vi "Update Actuator Setpoint.vi"(8 "error in (no error)":errorcluster, 11 "Model in":refnum<class "Model.lvclass">) -> (0 "error out":errorcluster, 3 "Model out":refnum<class "Model.lvclass">)   [LabVIEW 2015, in "Model.lvclass"]
uses:
  Model.lvclass
  Common_RT_FAILC/FAILC/FAILC.lvclass
  Modbus/DesktopModbus/DesktopModbus.lvclass
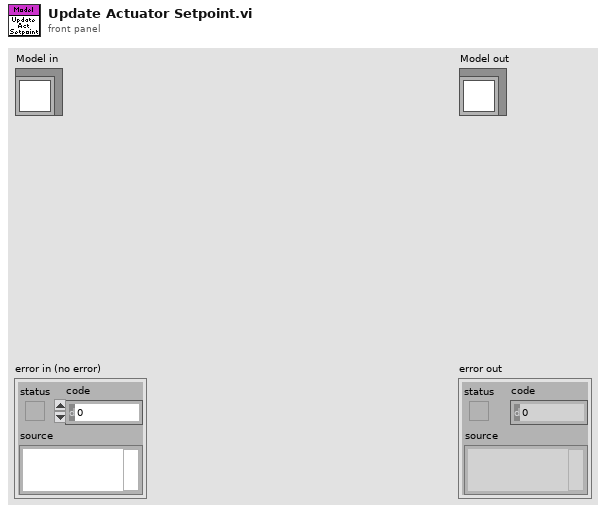
[diagram p1: front panel]
types:
  T1 = typedef "RTFAILC.lvlib/FAData.ctl" = cluster{"FAConstants":T2, "FACommand":T3, "FATelemetry":T5, "FAResponses":T6}
  T2 = typedef "RTFAILC.lvlib/FAConstants.ctl" = cluster{"ID":i16}
  T3 = typedef "RTFAILC.lvlib/FACommand.ctl" = cluster{"AxialSetPoint":i32, "LateralSetPoint":i32, "PressureServoValveSettings":T4, "BoosterValveSettings":T4}
  T4 = typedef "RTFAILC.lvlib/FAPID.ctl" = cluster{"Kp":sgl, "Ki":sgl, "Kd":sgl, "Kf":sgl}
  T5 = typedef "RTFAILC.lvlib/FATelemetry.ctl" = cluster{"ILCFault":bool, "BroadcastCounter":u8, "AxialLoadCellForce":sgl, "LateralLoadCellForce":sgl, "AxialPressure":T4, "AxialTurbo":T4, "LateralPressure":T4, "LateralTurbo":T4}
  T6 = typedef "RTFAILC.lvlib/FAResponses.ctl" = cluster{"PIDParameters":T7, "ReadPIDParameters":T7, "SetForce":T7, "ForceAndStatus":T7}
  T7 = typedef "RTModbus.lvlib/ExceptionCodes.ctl" = u16
  T8 = typedef "RTModbus.lvlib/Frame.ctl" = cluster{"Data":u8[], "WaitForTrigger":bool, "WaitForRx":u16, "TriggerIRQ":bool, "DelayTicks":u16, "DelayMicroseconds":u16, "DelayMilliseconds":u16}
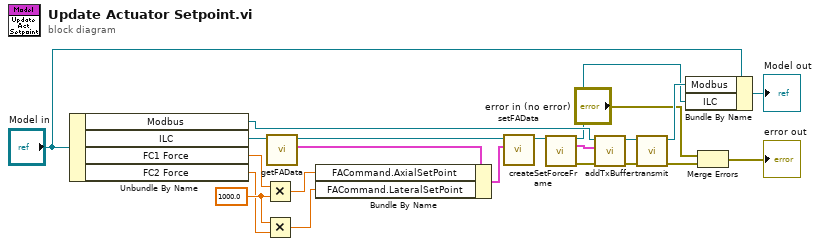
[diagram p0: block diagram]
diagram:
  w17 = 1000.0 ("y")
  n1 = Unbundle By Name("Model in") -> ("Modbus"=w9:refnum<class "DesktopModbus.lvclass">, "ILC"=w12:refnum<class "FAILC.lvclass">, "FC1 Force"=w19:dbl, "FC2 Force"=w16:dbl)
  n2 = Multiply(x=w19, y=w17) -> (x*y=w18:dbl)
  n3 = Multiply(x=w17, y=w16) -> (x*y=w15:dbl)
  n4 = call "getFAData.vi"("FAILC in"=w12) -> ("FAData"=w20:T1, "FAILC out"=w13:refnum<class "FAILC.lvclass">)  [unwired: 9 in]
  n5 = Bundle By Name(cluster=w20, "FACommand.AxialSetPoint"=w18, "FACommand.LateralSetPoint"=w15) -> (w14:T1)
  n6 = call "setFAData.vi"("FAData"=w14, "FAILC in"=w13) -> ("FAILC out"=w11:refnum<class "FAILC.lvclass">)  [unwired: 9 in]
  n7 = call-dynamic "createSetForceFrame.vi"("FAILC in"=w11) -> ("FAILC out"=w4:refnum<class "FAILC.lvclass">, "Frame"=w8:T8, "error out"=w7:errorcluster)  [unwired: 12 in]
  n8 = call-dynamic "addTxBuffer.vi"("error in (no error)"=w7, "Frame"=w8, "DesktopModbus in"=w9) -> ("error out"=w6:errorcluster, "DesktopModbus out"=w10:refnum<class "DesktopModbus.lvclass">)  [unwired: 7 in]
  n9 = call-dynamic "transmit.vi"("error in (no error)"=w6, "DesktopModbus in"=w10) -> ("error out"=w3:errorcluster, "DesktopModbus out"=w5:refnum<class "DesktopModbus.lvclass">)  [unwired: 8 in]
  n10 = Bundle By Name(cluster="Model in", "Modbus"=w5, "ILC"=w4) -> (→"Model out":refnum<class "Model.lvclass">)
  n11 = Merge Errors("error in (no error)", w3) -> (→"error out":errorcluster)
